vi "NewCombined.vi"() -> ()   [LabVIEW 2020]
uses:
  Stage/New/StageOptions.ctl
  Stage/New/SettingCtrlOptions.ctl
  Stage/New/PosCtrlOptions.ctl
  Stage/libximc.lvlib
  <instrlib>/_niInstr/Basic Elements/v1/FPGA/niInstr Basic Elements v1 FPGA.lvlib
  Digi/Digitizer_StatesMain.ctl
  Digi/SubVIs/DigiFPGARef.ctl
  <vilib>/rvi/interface/nirviMethod/nirviMethod.xnode
  <vilib>/FPGAPlugInAG/Dynamic/niLvFpga_Reset_Dynamic.vi
  <vilib>/rvi/interface/nirviReadWriteControl/nirviReadWriteControl.xnode
  NiFpgaLv.dll
  <vilib>/Utility/error.llb/Error Cluster From Error Code.vi
  <vilib>/rvi/interface/Simulation/niFpgaSimulationCallBeginRW.vi
  <vilib>/rvi/errors/niLvFpgaAdjustHostInterfaceError.vi
  <vilib>/rvi/interface/nirviCloseFPGA/nirviCloseFPGA.xnode
  <vilib>/FPGAPlugInAG/Dynamic/niLvFpga_Close_Dynamic.vi
  Gen/Generator_States.ctl
  ScanStates_main.ctl
  <vilib>/UPVI/lvhdf5/file.llb/LVH5F Operation.ctl
  <vilib>/UPVI/lvhdf5/dataset.llb/LVH5D Operation.ctl
  <vilib>/UPVI/lvhdf5/library.llb/HDF5 Ref.ctl
  <vilib>/Utility/miscctls.llb/LVRectTypeDef.ctl
  <vilib>/UPVI/lvhdf5/identifier.llb/Not an HDF5 Refnum Constant.vi
  <vilib>/UPVI/lvhdf5/dataset.llb/Simple H5Dwrite (Variant).vi
  <vilib>/UPVI/lvhdf5/dataset.llb/OpenCreateReplace Dataset by Element Type.vi
  <vilib>/UPVI/lvhdf5/dataspace.llb/H5Sselect_hyperslab.vi
  <vilib>/UPVI/lvhdf5/dataset.llb/H5Dwrite (Variant).vi
  <vilib>/UPVI/lvhdf5/dataset.llb/H5Dget_space.vi
  <vilib>/UPVI/lvhdf5/attribute.llb/private/LVH5AwriteWDTAttrs.vi
  <vilib>/UPVI/lvhdf5/dataspace.llb/H5Sclose.vi
  <vilib>/UPVI/lvhdf5/group.llb/H5G_obj_t.ctl
  <vilib>/UPVI/lvhdf5/utility.llb/Select HDF5 Dialog.vi
  <vilib>/UPVI/lvhdf5/dataset.llb/Simple H5Dwrite.xnode
  <vilib>/UPVI/lvhdf5/dataset.llb/Append Element(s) to Dataset (Variant).vi
  <vilib>/UPVI/lvhdf5/dataset.llb/Append Element(s) to Dataset.xnode
  <instrlib>/_niInstr/Basic Elements/v1/FPGA/Private/Count Up U32.vi
  <vilib>/UPVI/lvhdf5/utility.llb/Select HDF5 Dialog (File and Object).vi
  <vilib>/UPVI/lvhdf5/utility.llb/Select HDF5 Dialog (Object Only).vi
  FileStore/H5_WriteAttr.vi
  Digi/Controls/FPGA VI Reference.ctl
  <vilib>/userdefined/High Color/nirio_resource_hc.ctl
panel:
  out "Gen State":T1
  in  "Send vi Trig":bool
  in  "Generator Resource":refnum<k15>
  in  "Use Default Wave Settings":bool caption="Checkbox"
  in  "Stop Generator \nApplication":bool
  out "Gain":dbl
  out "Offset Factor":dbl
  out "Amplitudes":dbl[](array[numeric]) format="%.2f"
  out "Sampling Frequency (Hz)":u64
  out "Waves per Pixel":u32
  in  "Ext/nViTrig":bool=TRUE
  out "Gen Actual Sample Rate":dbl format="%#_6p"
  in  "Start Gen":bool
  in  "stop Gen":bool
  out "Generator On":bool
  out "Input Waveform":dbl[](graph)
  out "Intensity Graph":dbl[][](graph)
  in  "File Directory":path
  in  "Filename":string
  in  "Start Scan":bool
  in  "TrigIn_Sim":bool caption="Pause"
  in  "Delay(us)":sgl min=0 step=0.1 format="%#_4g"
  in  "Record Size":u16=1024
  in  "Time Division":u8(slide)=1 max=2 step=1 scale=0.0..2.0
  in  "Amplitude \nAveraging":u16(slide)=1 caption="Amplitude Averaging" scale=0.0..8.0 scale format="%#.2g"
  out "Configured?":bool
  out "TIS Configured?":bool
  in  "Start Digi":bool
  out "Digitizer On":bool
  in  "FineDelay  Control":dbl(slide)=1.0 scale=-2.0..2.0
  in  "Amplitude Range":cluster{"Slider 1":dbl, "Slider 1":dbl}(slide)={"Slider 1"=1.0, "Slider 1"=1.6299559471365639} scale=-2.5..2.5
  in  "Range":dbl=2.0
  out "Waveform LIVE":cluster{"Start Time":dbl, dbl, ext[]}(graph)
  out "Trigger Count":u32
  in  "reset":bool
  out "count out":u32
  out "Trig In":u32
  in  "Trigger Type":enum8{"Software", "Data Edge"}(ring)
  out "AvgCount_powerOf2":u16(knob) caption="Amplitude Avg" max=8 step=1 scale=0.0..8.0
  out "WaveSampleCount":i16=1024
  in  "Trigger Level (V)":dbl
  out "Read Size (Host)":u16
  out "TimeDivFactor":i16
  out "FPGA VI Reference Out":T2
  out "range (Vpp)":dbl=1.3
  out "Digi State":T3
  in  "Machine Mode":T4(ring)=enum."Normal"
  in  "nGenTrig/vi":bool=TRUE caption="Trigger Mode"
  in  "Digi RIO Resource":T5="PXI1Slot2"
  in  "Stop Digi App":bool caption="Stop Digi \nApplication"
  out "Moving?":bool
  out "Stage Position":cluster{sgl[], sgl[]}(graph) caption="XY Graph - Dark"
  in  "X Position Abs":dbl caption="X Position"
  in  "Y Position Abs":dbl caption="Y Position"
  out "Line Count":i32=6
  out "Pixel Count":i32=6
  in  "X Start":sgl
  in  "X End":sgl=10.0
  in  "Y Start":sgl
  in  "Y End":sgl=8.0
  in  "Y Step Size 2":sgl=0.5
  in  "X Step Size 2":sgl=0.5
  in  "Scan Mode":enum16{"Raster", "Serpentine"}(ring)
  out "X Step Size":sgl format="%#.2g"
  out "Y Step Size":sgl format="%#.2g"
  in  "Speed Control (mm/s)":sgl(slide)=1.0 min=0.1 scale=0.1..5.0
  in  "AbsMove":bool
  in  "Outline":bool
  in  "Start Stage":bool
  in  "Stop Motion":bool
  in  "Zero":bool
  in  "Right":bool
  in  "Left":bool
  in  "Move to Start":bool
  in  "Down":bool
  in  "Up":bool
  out "X Position":dbl format="%#.3g"
  out "Y Position":dbl format="%#.3g"
  in  "Move Step":dbl=1.0
  in  "Stop Stage":bool
  out "Controller Open?":bool
  in  "Next Coordinate Index":i32
  out "Coordinate Array":sgl[][](array[numeric])
  out "Step Sizes":sgl[](array[numeric])
  out "Peripheral Coordis":sgl[][](array[numeric])=[[0.0, 0.0], [1.8, 0.0], [3.6, 0.0], [5.3999996, 0.0], [7.2, 0.0], [9.0, 0.0], [9.0, 2.0], [7.2, 2.0], [5.3999996, 2.0], [3.6, 2.0], [1.8, 2.0], [0.0, 2.0], [0.0, 4.0], [1.8, 4.0], [3.6, 4.0], [5.3999996, 4.0], [7.2, 4.0], [9.0, 4.0], [9.0, 6.0], [7.2, 6.0], [5.3999996, 6.0], [3.6, 6.0], [1.8, 6.0], [0.0, 6.0], [0.0, 8.0], [1.8, 8.0], [3.6, 8.0], [5.3999996, 8.0], [7.2, 8.0], [9.0, 8.0], [9.0, 10.0], [7.2, 10.0], [5.3999996, 10.0], [3.6, 10.0], [1.8, 10.0], [0.0, 10.0]]
  out "Serial nos":u32[](array[numeric])
  out "Calibration":cluster{dbl, "MicrostepMode":u32}[](array[cluster])
  out "IDs":i32[](array[numeric])
  out "Move Step halved":dbl=1.0
  out "X Max Stage":dbl=220.0 format="%#_13g"
  out "Y Maximum":dbl
  in  "Correction Table Path (Hidden)":path
  in  "EdgePt/nPixelMap":bool=TRUE
  out "Stage Status":T6
  in  "Close Stage":bool
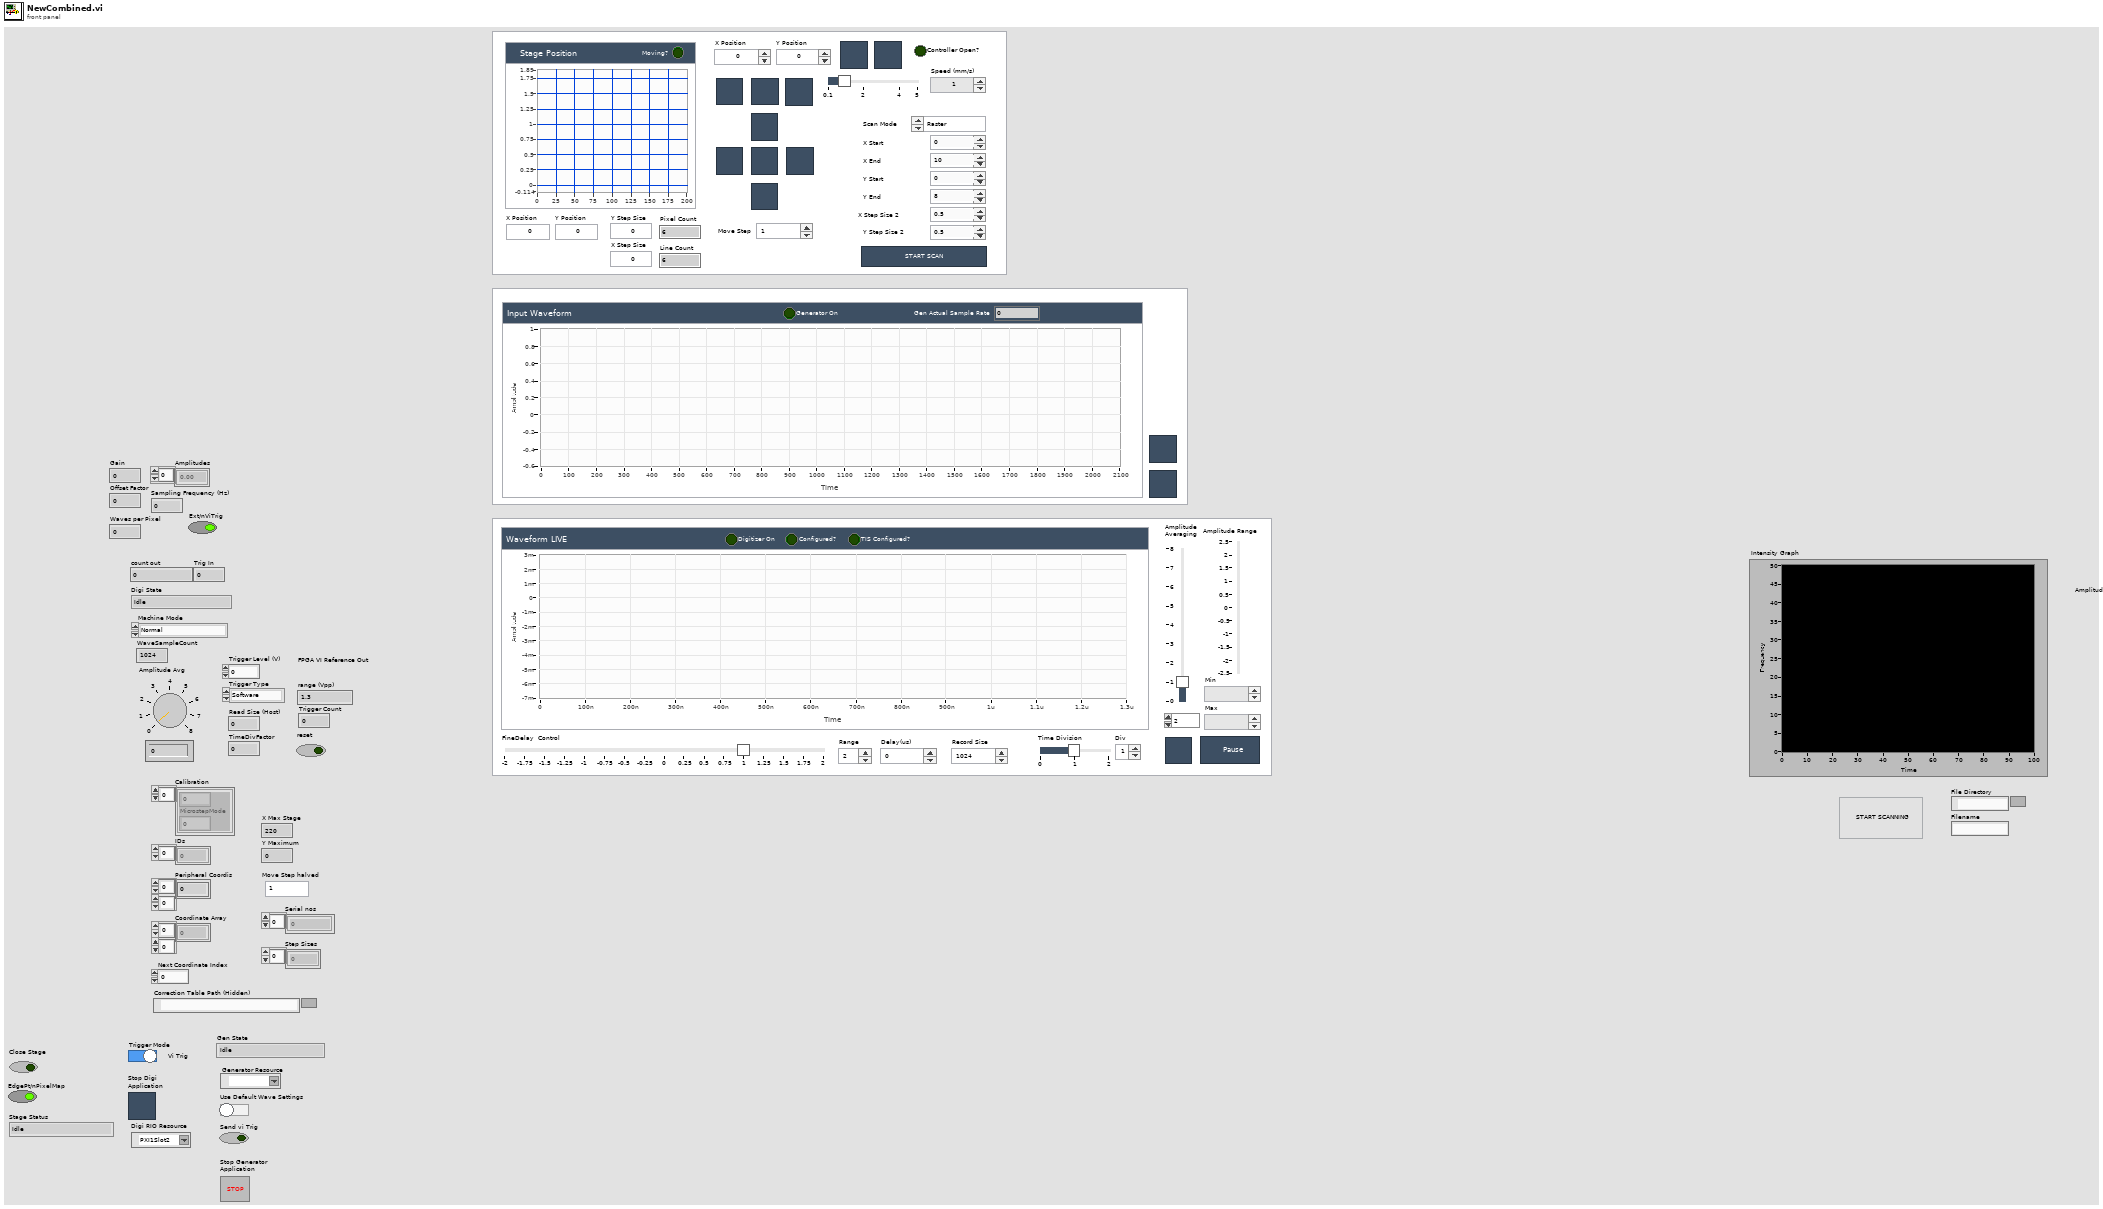
[diagram p1: front panel]
types:
  T1 = typedef "Generator_States.ctl" = enum16{"Idle", "GenerateWaveArray", "InitGen", "SendVITrig", "CloseGen", "CloseApp"}
  T2 = typedef "DigiFPGARef.ctl" = refnum<k20>
  T3 = typedef "Digitizer_StatesMain.ctl" = enum16{"Idle", "Init", "SetParam", "VITrig", "Read", "CloseDigi", "CloseApp"}
  T4 = enum16{"Scanning Mode", "Perimeter Mode", "Normal"}
  T5 = typedef "nirio_resource_hc.ctl" = tag
  T6 = typedef "StageOptions.ctl" = enum16{"Idle", "Init", "Set Speed", "GenerateMotionPoints", "Scan_Start", "Scan_MoveNext", "Scan_SyncSet", "Scan_Get Pos", "Scan_Complete", "Cmd_MoveAbs", "Cmd_CloseControllers", "Cmd_MoveUp", "Cmd_MoveDown", "Cmd_MoveLeft", "Cmd_MoveRight", "Cmd_MoveStart", "Cmd_MoveZero", "Cmd_GetPos", "Cmd_Stop", "Sync_On", "Sync_Off", "Stop Motion", "CloseApplication"}
  T7 = typedef "ScanStates_main.ctl" = enum16{"Idle", "Init", "Get Data", "Store Data", "Close Files"}
  T8 = typedef "SettingCtrlOptions.ctl" = enum16{"Set X", "Set Y", "Set X and Y", "Get Settings", "None"}
  T9 = typedef "PosCtrlOptions.ctl" = enum16{"Move X", "Move Y", "Both X and Y", "Read Pos", "None"}
  T10 = typedef "FPGA VI Reference.ctl" = refnum<k20>
  T11 = typedef "LVH5D Operation.ctl" = enum16{"open", "replace", "create", "open or create", "create or replace", "create or replace with confirmation"}
  T12 = typedef "LVH5F Operation.ctl" = enum16{"open", "open or create", "create or replace", "create or replace (with confirmation)", "create", "open (read only)"}
  T13 = typedef "LVRectTypeDef.ctl" = cluster{"Left":i16, "Top":i16, "Right":i16, "Bottom":i16}
  T14 = cluster{"Behavior":enum32{"Invalid", "Default", "Floating", "Floating/Auto-Hide", "Modal"}, "Position":T13, "Center":bool, "Title":string}
  T15 = typedef "H5G_obj_t.ctl" = i32
  T16 = cluster{"Object Types (any)":T15[], "Object Pattern":string}
  T17 = typedef "HDF5 Ref.ctl" = refnum<k1>
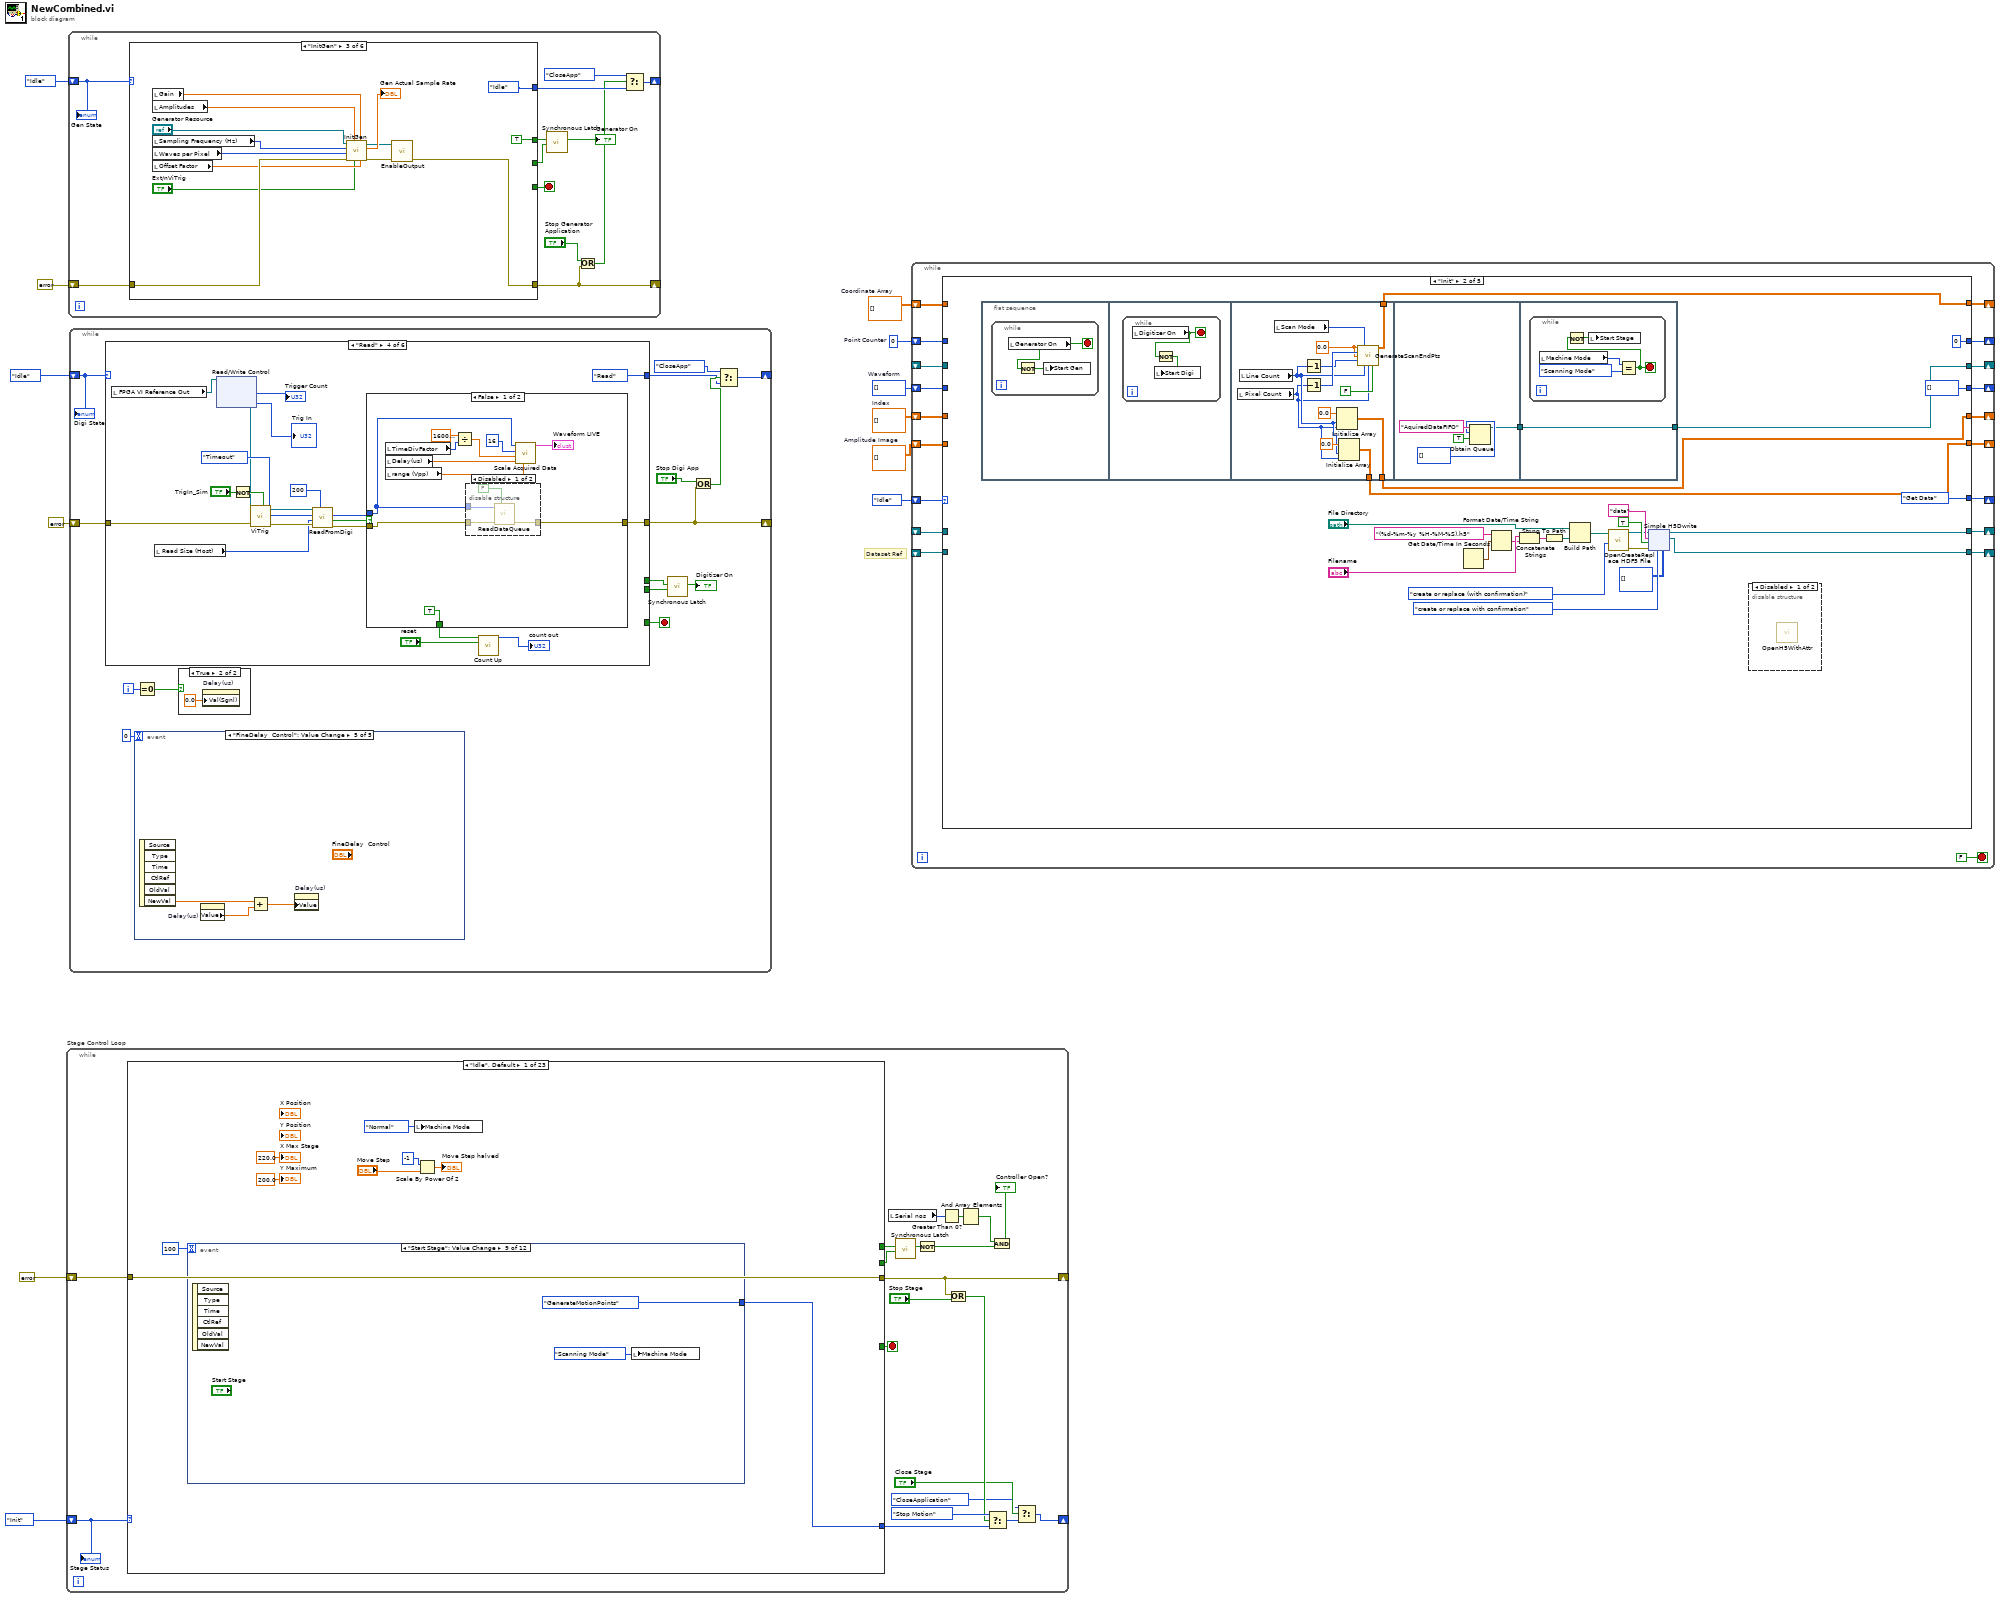
[diagram p0: block diagram]
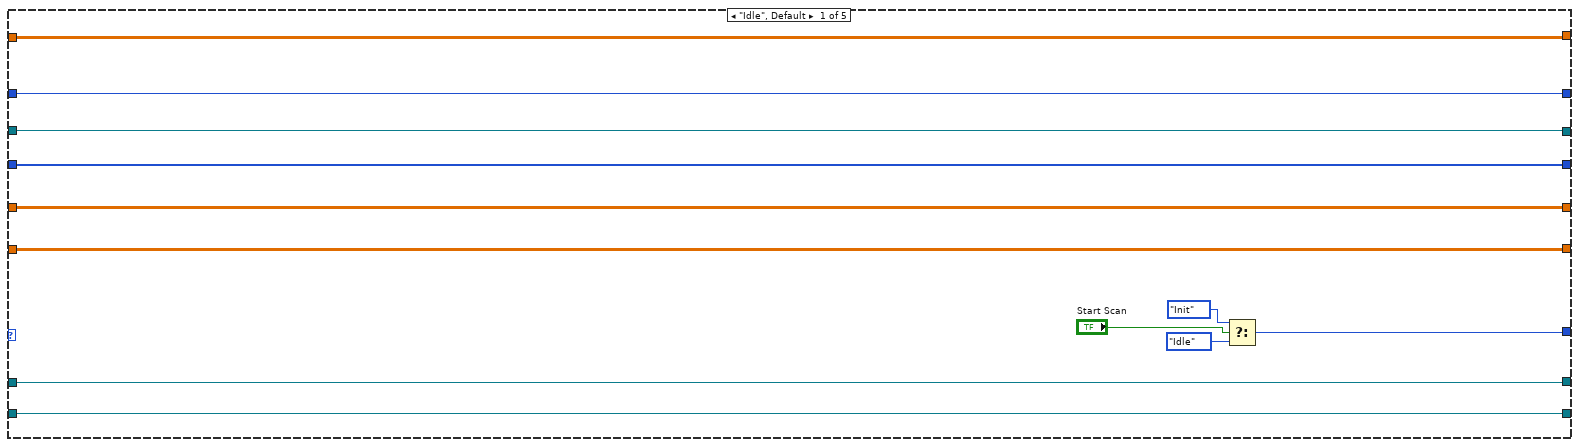
[diagram p2: hidden frame]
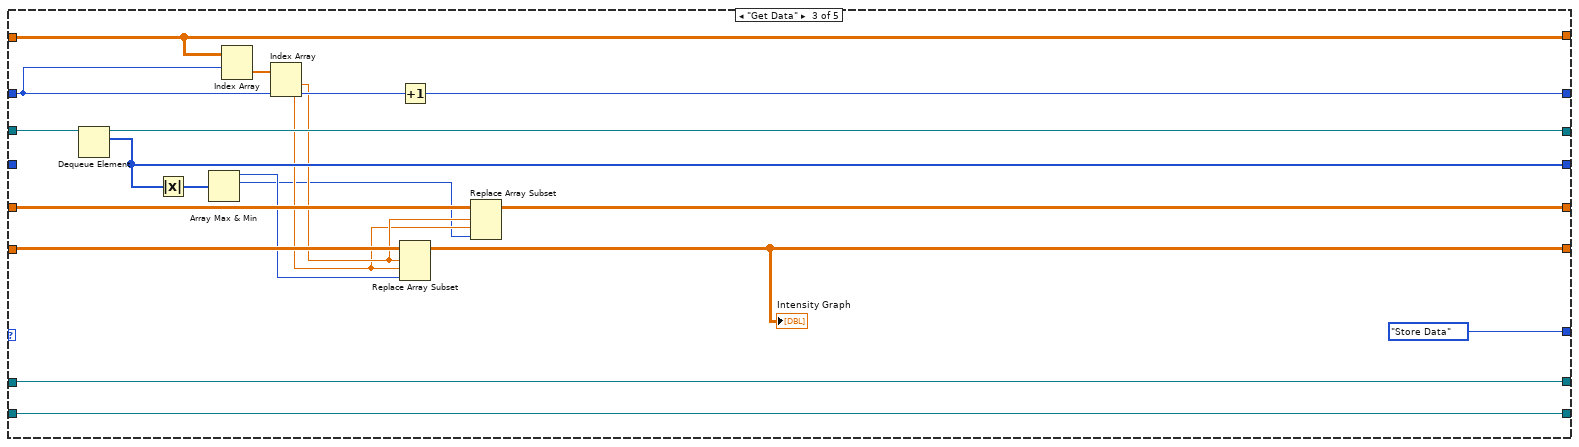
[diagram p4: hidden frame]
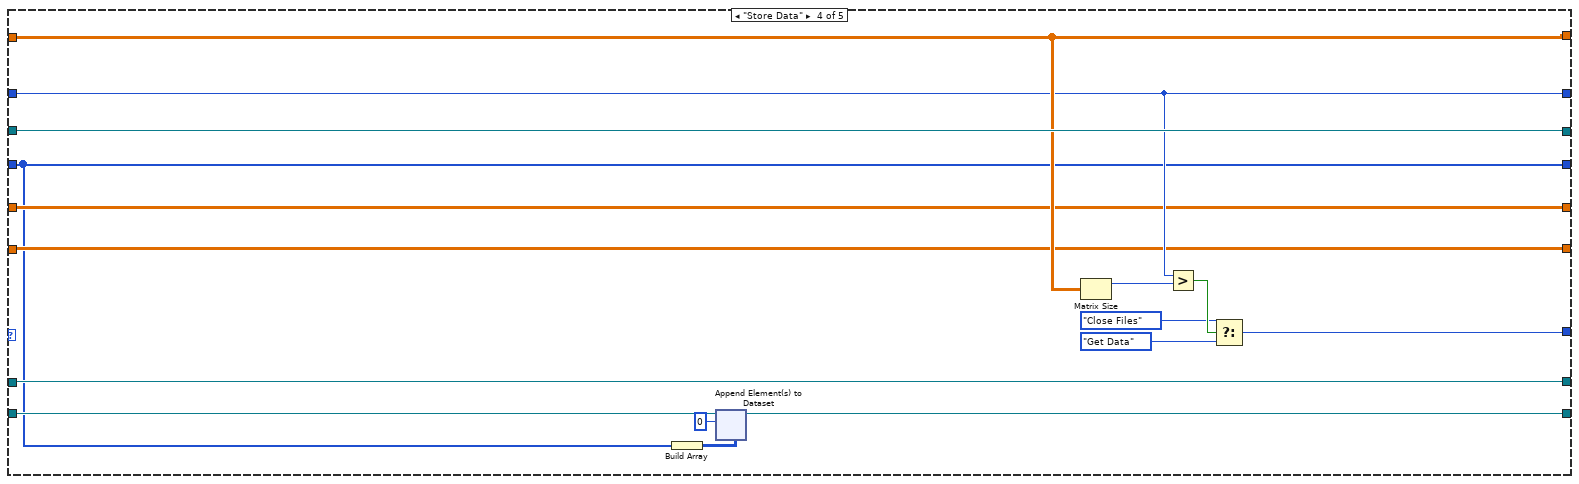
[diagram p5: hidden frame]
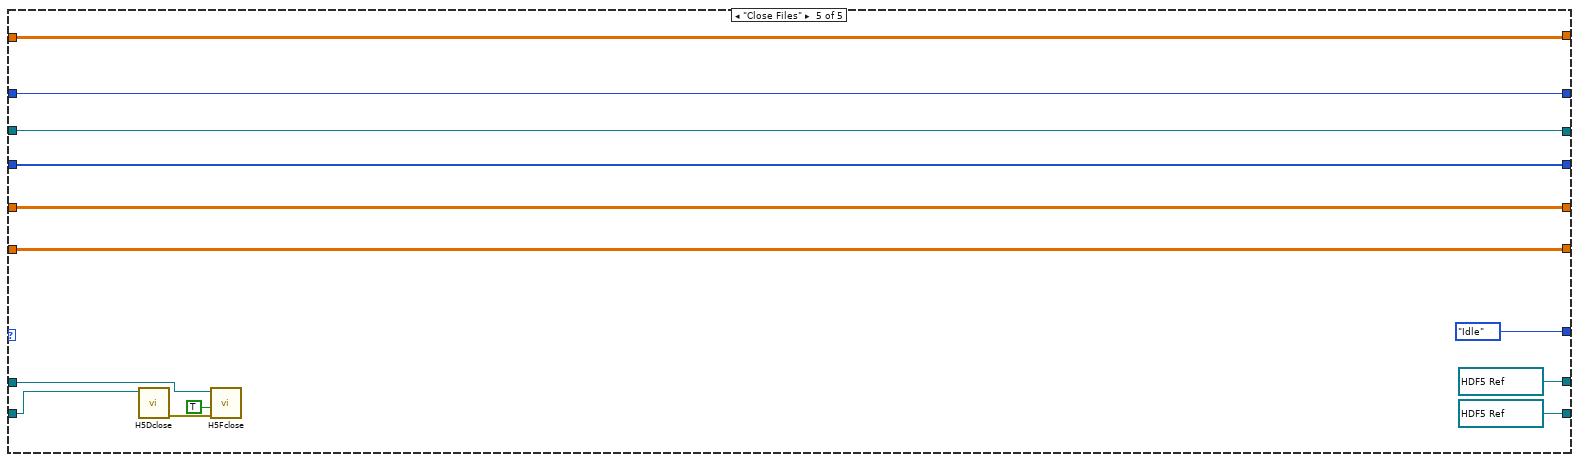
[diagram p6: hidden frame]
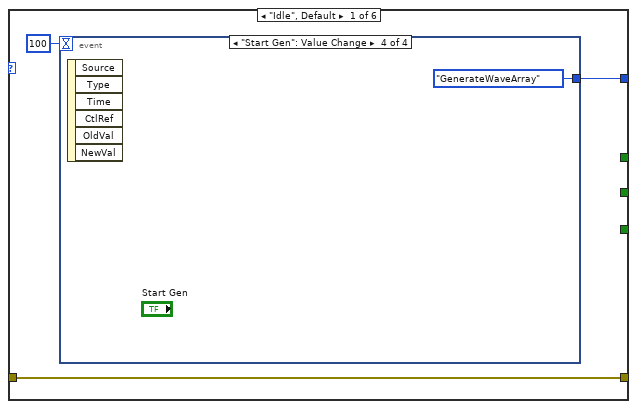
[diagram p7: hidden frame]
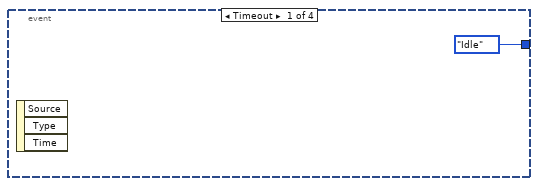
[diagram p8: hidden frame]
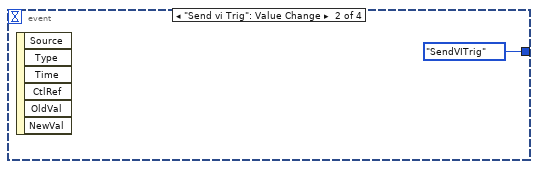
[diagram p9: hidden frame]
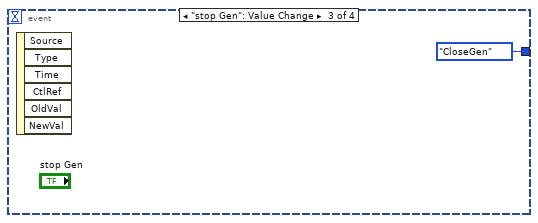
[diagram p10: hidden frame]
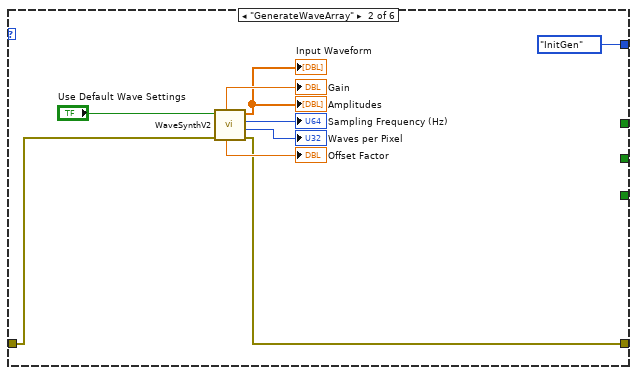
[diagram p11: hidden frame]
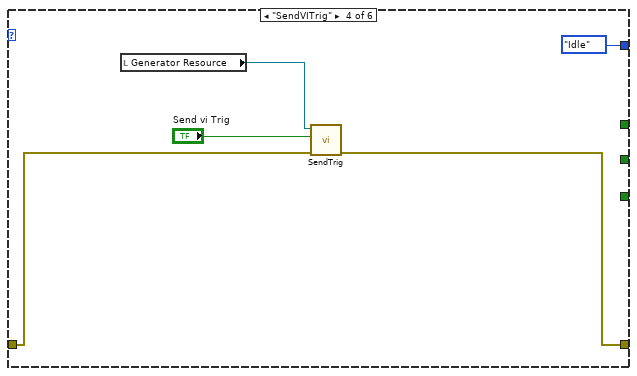
[diagram p12: hidden frame]
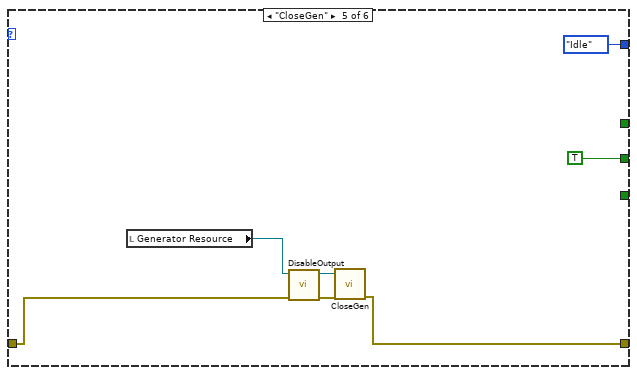
[diagram p13: hidden frame]
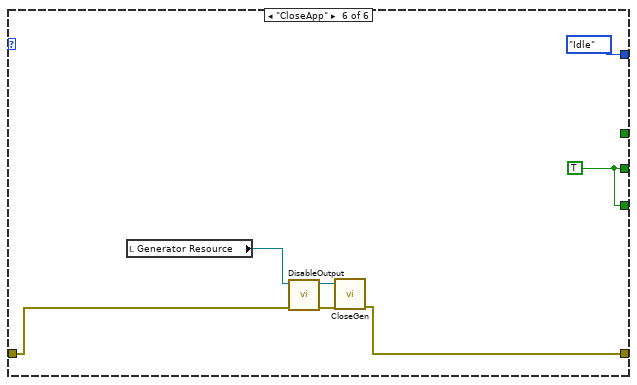
[diagram p14: hidden frame]
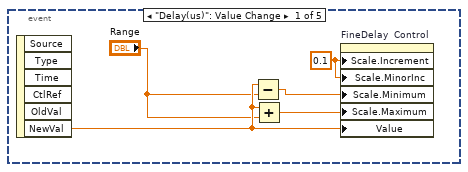
[diagram p15: hidden frame]
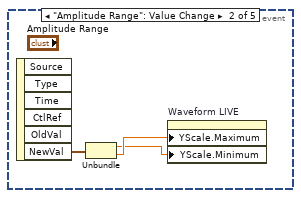
[diagram p16: hidden frame]
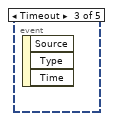
[diagram p17: hidden frame]
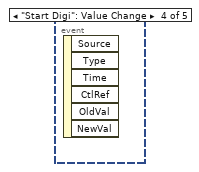
[diagram p18: hidden frame]
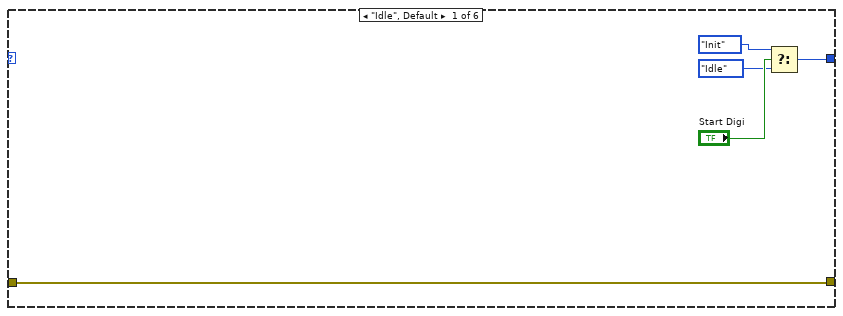
[diagram p20: hidden frame]
diagram:
  w6 = dbl[][] []  # Index
  w5 = dbl[][] []  # Amplitude Image
  w4 = i16[] []  # Waveform
  w3 = sgl[][] []  # Coordinate Array
  w2 = u64 0  # Point Counter
  # "Dataset Ref"
  n1 = while "Stage Control Loop" {
    shift-right: [w21] -> _
    shift-left: StageOptions."Init" -> [w32]
    shift-right: [w29] -> _
    shift-left: errorcluster {"status"=FALSE, "code"=0, "source"=""} ("error out") -> [w30]
    stop <- w22 stop-if-true
    n2 = case shown="\"Idle\", Default" w32 {
      tunnel: [w41 w82 w105 w134 w148 w180 w194 w207 w248 w257 w266 w273 w284 w294 w304 w313 w321 w336 w342 w353 w362 w369 w379] -> w29
      tunnel: w30 -> [w41 w89 w106 w133 w154 w181 w195 w208 w249 w258 w267 w272 w285 w295 w305 w314 w322 w337 w341 w354 w363 w368 w378]
      tunnel: [w40 StageOptions."Set Speed" StageOptions."Idle" w114 StageOptions."Scan_Get Pos" w169 StageOptions."Scan_MoveNext" w204 StageOptions."Idle" StageOptions."Idle" StageOptions."Idle" StageOptions."Idle" StageOptions."Idle" StageOptions."Idle" StageOptions."Idle" StageOptions."Idle" StageOptions."Idle" StageOptions."Idle" StageOptions."Idle" StageOptions."Idle" StageOptions."Idle" StageOptions."Idle" StageOptions."Idle"] -> w27
      tunnel: [_ _ _ _ _ _ _ _ _ _ _ _ _ _ _ _ _ _ _ _ _ w365 w374] -> w25
      tunnel: [_ w83 _ _ _ _ _ _ _ _ _ _ _ _ _ _ _ _ _ _ _ _ _] -> w23
      tunnel: [_ _ _ _ _ _ _ _ _ _ _ _ _ _ _ _ _ _ _ _ _ _ w374] -> w22
      frame "Idle", Default {
        n3 = event shown="[8] \"Start Stage\": Value Change" {
          selector: _ -> [_ _ _ _ _ _ _ _ _ _ _ _]
          dyn-events: _ -> [_ _ _ _ _ _ _ _ _ _ _ _]
          timeout: 100 -> [_ _ _ _ _ _ _ _ _ _ _ _]
          tunnel: [w42 StageOptions."Cmd_MoveUp" StageOptions."Cmd_MoveDown" StageOptions."Cmd_MoveStart" StageOptions."Cmd_MoveLeft" StageOptions."Cmd_MoveRight" StageOptions."Cmd_MoveZero" StageOptions."Cmd_Stop" StageOptions."GenerateMotionPoints" StageOptions."Set Speed" w77 StageOptions."Cmd_MoveAbs"] -> w40
          event Timeout {
            n4 = event-data() -> ()  [unwired: 1 in, 3 out]
            n5 = local read "Controller Open?"() -> (w43:bool)
            n6 = case shown="True" w43 {
              tunnel: [StageOptions."Init" StageOptions."Cmd_GetPos"] -> w42
              frame False {
              }
              frame True {
              }
            }
          }
          event "Up": Value Change {
            w48 = 0.0 ("X Scale.Range:Minimum")
            n7 = event-data() -> ()  [unwired: 1 in, 6 out]
            n8 = local read "X Max Stage"() -> (w47:dbl)
            n9 = local read "Y Maximum"() -> (w46:dbl)
            n10 = Build Array(w48, w47) -> (w50:dbl[])
            n11 = Build Array(w48, w46) -> (w49:dbl[])
            n12 = property on="Stage Position" class="XYGraph (strict)"("XScale.Maximum"=w47, "XScale.Minimum"=w48, "YScale.Maximum"=w46, "YScale.Minimum"=w48, "XScale.MarkerVals[]"=w50, "YScale.MarkerVals[]"=w49) -> ()  [unwired: 2 in, 2 out]
          }
          event "Down": Value Change {
            w54 = 0.0 ("X Scale.Range:Minimum")
            n13 = event-data() -> ()  [unwired: 1 in, 6 out]
            n14 = local read "X Max Stage"() -> (w53:dbl)
            n15 = local read "Y Maximum"() -> (w52:dbl)
            n16 = Build Array(w54, w53) -> (w56:dbl[])
            n17 = Build Array(w54, w52) -> (w55:dbl[])
            n18 = property on="Stage Position" class="XYGraph (strict)"("XScale.Maximum"=w53, "XScale.Minimum"=w54, "YScale.Maximum"=w52, "YScale.Minimum"=w54, "XScale.MarkerVals[]"=w56, "YScale.MarkerVals[]"=w55) -> ()  [unwired: 2 in, 2 out]
          }
          event "Move to Start": Value Change {
            n19 = event-data() -> ()  [unwired: 1 in, 6 out]
          }
          event "Left": Value Change {
            w61 = 0.0 ("X Scale.Range:Minimum")
            n20 = event-data() -> ()  [unwired: 1 in, 6 out]
            n21 = local read "X Max Stage"() -> (w60:dbl)
            n22 = local read "Y Maximum"() -> (w59:dbl)
            n23 = Build Array(w61, w60) -> (w63:dbl[])
            n24 = Build Array(w61, w59) -> (w62:dbl[])
            n25 = property on="Stage Position" class="XYGraph (strict)"("XScale.Maximum"=w60, "XScale.Minimum"=w61, "YScale.Maximum"=w59, "YScale.Minimum"=w61, "XScale.MarkerVals[]"=w63, "YScale.MarkerVals[]"=w62) -> ()  [unwired: 2 in, 2 out]
          }
          event "Right": Value Change {
            w65 = 0.0 ("X Scale.Range:Minimum")
            n26 = event-data() -> ()  [unwired: 1 in, 6 out]
            n27 = local read "X Max Stage"() -> (w67:dbl)
            n28 = local read "Y Maximum"() -> (w66:dbl)
            n29 = Build Array(w65, w67) -> (w69:dbl[])
            n30 = Build Array(w65, w66) -> (w68:dbl[])
            n31 = property on="Stage Position" class="XYGraph (strict)"("XScale.Maximum"=w67, "XScale.Minimum"=w65, "YScale.Maximum"=w66, "YScale.Minimum"=w65, "XScale.MarkerVals[]"=w69, "YScale.MarkerVals[]"=w68) -> ()  [unwired: 2 in, 2 out]
          }
          event "Zero": Value Change {
            n32 = event-data() -> ()  [unwired: 1 in, 6 out]
          }
          event "Stop Motion": Value Change {
            n33 = event-data() -> ()  [unwired: 1 in, 6 out]
          }
          event "Start Stage": Value Change {
            n34 = event-data() -> ()  [unwired: 1 in, 6 out]
            n35 = local write "Machine Mode"(T4."Scanning Mode" ("Machine Mode")) -> ()
          }
          event "Speed Control (mm/s)": Value Change {
            n36 = event-data() -> ()  [unwired: 1 in, 6 out]
          }
          event "Outline": Value Change {
            n37 = event-data() -> ()  [unwired: 1 in, 6 out]
            n38 = case shown="False" "Outline" {
              tunnel: [StageOptions."Idle" StageOptions."GenerateMotionPoints"] -> w77
              frame False {
              }
              frame True {
                n39 = local write "Machine Mode"(T4."Perimeter Mode" ("Machine Mode")) -> ()
              }
            }
          }
          event "AbsMove": Value Change {
            n40 = event-data() -> ()  [unwired: 1 in, 6 out]
          }
        }
        n41 = local write "Machine Mode"(T4."Normal" ("Machine Mode")) -> ()
        n42 = Scale By Power Of 2(n=i16 -1, x="Move Step") -> (x*2^n=→"Move Step halved":dbl)
        "X Max Stage" <- 220.0 ("X Max Stage")
        "Y Maximum" <- 200.0 ("Y Maximum")
      }
      frame "Init" {
        w90 = 100  # numSteps = 1mm
        w91 = TRUE  # Correction File Path Option
        n43 = case shown="False" w91 {
          tunnel: ["Correction Table Path (Hidden)" w97] -> w92
          frame False {
          }
          frame True {
            w98 = path "Corr_table_8MT173-25.tbl"  # File Name
            n44 = Current VI's Path() -> (path=w100:path)
            n45 = Build Path(base path=w100, name or relative path=path "") -> (appended path=w99:path)
            n46 = Build Path(base path=w99, name or relative path=w98) -> (appended path=w97:path)
          }
        }
        n47 = call "Find Controllers.vi"("error in (no error)"=w89) -> ("error out"=w94:errorcluster, "Names"=w95:string[])  [unwired: 8 in, 1 out]
        n48 = call "OpenDevices.vi"("error In"=w94, "Names"=w95) -> ("error out"=w93:errorcluster, "Serial nos"=→"Serial nos":u32[], "IDs"=w87:i32[])  [unwired: 6 in]
        "IDs" <- w87
        n49 = call "CalibrateStage.vi"("error in (no error)"=w93, "numSteps = 1mm"=w90, "Correction Table Path"=w92, "IDs"=w87) -> ("error out"=w82:errorcluster, "Calibration"=→"Calibration":cluster{dbl, "MicrostepMode":u32}[])  [unwired: 2 in, 4 out]
        n50 = Unbundle By Name(w82) -> ("status"=w84:bool)
        n51 = Not(x=w84) -> (.not. x?=w83:bool)
      }
      frame "Set Speed" {
        n52 = local read "IDs"() -> (w104:i32[])
        n53 = local read "Calibration"() -> (w103:cluster{dbl, "MicrostepMode":u32}[])
        n54 = call "SetMoveSettings.vi"("Mode"=SettingCtrlOptions."Set X and Y", "error in (no error)"=w106, "Calibration"=w103, "Speed"="Speed Control (mm/s)", "IDs"=w104) -> ("error out"=w105:errorcluster)  [unwired: 4 in, 2 out]
      }
      frame "GenerateMotionPoints" {
        n55 = local read "Calibration"() -> (w120:cluster{dbl, "MicrostepMode":u32}[])
        n56 = Subtract(x="X End", y="X Start") -> (x-y=w130:sgl)
        n57 = Increment(x=w130) -> (x+1=w129:sgl)
        n58 = Divide(x=w129, y="X Step Size 2") -> (x/y=w127:sgl)
        n59 = To Long Integer(number=w127) -> (32bit integer=w126:i32)
        "Pixel Count" <- w126
        n60 = Subtract(x="Y End", y="Y Start") -> (x-y=w124:sgl)
        n61 = Increment(x=w124) -> (x+1=w125:sgl)
        n62 = Divide(x=w125, y="Y Step Size 2") -> (x/y=w122:sgl)
        n63 = To Long Integer(number=w122) -> (32bit integer=w121:i32)
        "Line Count" <- w121
        n64 = call "GenerateScanEndPts.vi"("X Start"="X Start", "Mode"="Scan Mode", "Calibration In"=w120, "X End"="X End", "Y Start"="Y Start", "Y End"="Y End", "error in"=w133, "Line Count"=w121, "Pixel Count"=w126, "EdgePt/nPixelMap"="EdgePt/nPixelMap") -> ("Coordinate Array"=→"Coordinate Array":sgl[][], "Step Sizes"=w111:sgl[], "error out"=w134:errorcluster)  [unwired: 1 in, 2 out]
        "Step Sizes" <- w111
        n65 = call "PeripheralCoordinates.vi"("Y End"="Y End", "Y Start"="Y Start", "X End"="X End", "X Start"="X Start") -> ("Coordinate Array"=→"Peripheral Coordis":sgl[][])  [unwired: 7 in]
        n66 = Index Array(array=w111) -> (element #1=→"X Step Size":sgl, element #2=→"Y Step Size":sgl)  [unwired: 2 in]
        n67 = case shown="\"Perimeter Mode\"" "Machine Mode" {
          tunnel: [StageOptions."Scan_Start" StageOptions."Scan_Start" StageOptions."Idle"] -> w114
          frame "Scanning Mode" {
          }
          frame "Perimeter Mode" {
          }
          frame "Normal", Default {
          }
        }
      }
      frame "Scan_Start" {
        w151 = 0.0 ("element")
        w160 = 1.0  # Offset
        # "Draw Markers To Indicate the Scan Area"
        n68 = property on="X End" class="DigNum (strict)"() -> ("Value"=w159:sgl)  [unwired: 2 in, 2 out]
        n69 = property on="X Start" class="DigNum (strict)"() -> ("Value"=w158:sgl)  [unwired: 2 in, 2 out]
        n70 = property on="Y End" class="DigNum (strict)"() -> ("Value"=w155:sgl)  [unwired: 2 in, 2 out]
        n71 = property on="Y Start" class="DigNum (strict)"() -> ("Value"=w157:sgl)  [unwired: 2 in, 2 out]
        n72 = Add(x=w160, y=w159) -> (x+y=w162:dbl)
        n73 = Subtract(x=w158, y=w160) -> (x-y=w163:dbl)
        n74 = Add(x=w155, y=w160) -> (x+y=w161:dbl)
        n75 = Subtract(x=w157, y=w160) -> (x-y=w156:dbl)
        n76 = Build Array(w158, w159) -> (w165:sgl[])
        n77 = Build Array(w157, w155) -> (w164:sgl[])
        n78 = property on="Stage Position" class="XYGraph (strict)"(error in=w154, "XScale.Maximum"=w162, "XScale.Minimum"=w163, "YScale.Maximum"=w161, "YScale.Minimum"=w156, "XScale.MarkerVals[]"=w165, "YScale.MarkerVals[]"=w164) -> (error out=w140:errorcluster)  [unwired: 1 in, 1 out]
        n79 = local read "EdgePt/nPixelMap"() -> (w144:bool)
        n80 = local read "IDs"() -> (w147:i32[])
        n81 = local read "Step Sizes"() -> (w145:sgl[])
        n82 = local read "Calibration"() -> (w146:cluster{dbl, "MicrostepMode":u32}[])
        n83 = call "SetSyncSettings.vi"("Periodic/nPointScan"=w144, "X SyncOut Enabled"=FALSE, "Y SyncOut Enabled"=FALSE, "error in (no error)"=w140, "Calibration"=w146, "Step Sizes(mm)"=w145, "IDs"=w147) -> ("error out"=w141:errorcluster)  [unwired: 3 in, 1 out]
        n84 = local write "Next Coordinate Index"(0 ("Next Coordinate Index")) -> ()
        n85 = local read "IDs"() -> (w149:i32[])
        n86 = local read "Calibration"() -> (w150:cluster{dbl, "MicrostepMode":u32}[])
        n87 = Build Array(w151, w151) -> (w152:dbl[])
        n88 = call "PositionControlRelative.vi"("Mode"=PosCtrlOptions."Both X and Y", "error in (no error)"=w141, "Calibration"=w150, "Move to"=w152, "IDs"=w149) -> ("error out"=w148:errorcluster)  [unwired: 4 in, 2 out]
      }
      frame "Scan_Get Pos" {
        n89 = local read "IDs"() -> (w178:i32[])
        n90 = local read "Calibration"() -> (w179:cluster{dbl, "MicrostepMode":u32}[])
        n91 = call "PositionControl.vi"("Mode"=PosCtrlOptions."Read Pos", "error in (no error)"=w181, "Calibration"=w179, "IDs"=w178) -> ("error out"=w180:errorcluster, "Moving?"=w168:bool, "Position"=w171:sgl[])  [unwired: 4 in, 1 out]
        n92 = local write "Moving?"(w168) -> ()
        n93 = Index Array(array=w171, index #1=0 ("index"), index #2=1 ("index")) -> (element #1=w175:sgl, element #2=w174:sgl)
        n94 = local write "X Position"(w175) -> ()
        n95 = local write "Y Position"(w174) -> ()
        n96 = Build Array(w175) -> (w176:sgl[])
        n97 = Build Array(w174) -> (w177:sgl[])
        n98 = Bundle(w176, w177) -> (w170:cluster{sgl[], sgl[]})  [unwired: 1 in]
        n99 = local write "Stage Position"(w170) -> ()
        n100 = Select(t=StageOptions."Scan_Get Pos", s=w168, f=StageOptions."Scan_SyncSet") -> (s? t:f=w169:T6)
      }
      frame "Scan_SyncSet" {
        n101 = local read "EdgePt/nPixelMap"() -> (w184:bool)
        n102 = local read "IDs"() -> (w192:i32[])
        n103 = local read "Step Sizes"() -> (w190:sgl[])
        n104 = local read "Calibration"() -> (w191:cluster{dbl, "MicrostepMode":u32}[])
        n105 = Quotient & Remainder(x="Next Coordinate Index", y=2) -> (x-y*floor(x/y)=w187:i32)  [unwired: 1 out]
        n106 = Not Equal To 0?(x=w187) -> (x != 0?=w185:bool)
        n107 = Compound Arithmetic op=OR(invert w184, w185) -> (w186:bool)
        n108 = call "SetSyncSettings.vi"("Periodic/nPointScan"=w184, "X SyncOut Enabled"=w186, "Y SyncOut Enabled"=FALSE, "error in (no error)"=w195, "Calibration"=w191, "Step Sizes(mm)"=w190, "IDs"=w192) -> ("error out"=w194:errorcluster)  [unwired: 3 in, 1 out]
      }
      frame "Scan_MoveNext" {
        n109 = flat-sequence {
          tunnel: w208 -> [w211]
          tunnel: [w211] -> w199
          tunnel: [w210] -> w198
          tunnel: [w209] -> w196
          tunnel: [w219] -> w206
          tunnel: [w216] -> w205
          tunnel: [w215] -> w201
          tunnel: w199 -> [w220]
          tunnel: w198 -> [w215]
          tunnel: [w214] -> w197
          tunnel: w196 -> [w214]
          tunnel: [w230] -> w200
          tunnel: [w231] -> w207
          tunnel: w197 -> [w223]
          tunnel: w201 -> [w227]
          tunnel: w205 -> [w228]
          tunnel: w206 -> [w231]
          frame #0 {
            n110 = local read "Machine Mode"() -> (w209:T4)
            n111 = case shown="\"Perimeter Mode\"" w209 {
              tunnel: [w212 w213] -> w210
              frame "Scanning Mode", Default {
                n112 = local read "Coordinate Array"() -> (w212:sgl[][])
              }
              frame "Perimeter Mode" {
                n113 = local read "Peripheral Coordis"() -> (w213:sgl[][])
              }
            }
          }
          frame #1 {
            n114 = local read "IDs"() -> (w218:i32[])
            n115 = local read "Next Coordinate Index"() -> (w216:i32)
            n116 = local read "Calibration"() -> (w217:cluster{dbl, "MicrostepMode":u32}[])
            n117 = Index Array(array=w215, index (row)=w216) -> (element=w221:sgl[])  [unwired: 1 in]
            n118 = call "PositionControl.vi"("Mode"=PosCtrlOptions."Both X and Y", "error in (no error)"=w220, "Calibration"=w217, "Move to"=w221, "IDs"=w218) -> ("error out"=w219:errorcluster)  [unwired: 3 in, 3 out]
          }
          frame #2 {
            n119 = Matrix Size(0:w227) -> (1:w226:i32)  [unwired: 1 out]
            n120 = Increment(x=w228) -> (x+1=w224:i32)
            n121 = Greater?(x=w224, y=w226) -> (0:w225:bool)
            n122 = case shown="True" w225 {
              selector: w225 -> [w232 _]
              tunnel: w224 -> [w233 w236]
              tunnel: [w233 w235] -> w229
              tunnel: [w232 w234] -> w230
              tunnel: w223 -> [_ w237]
              frame False {
              }
              frame True {
                n123 = case shown="\"Scanning Mode\", Default" w237 {
                  tunnel: w236 -> [w239 _]
                  tunnel: [w239 0] -> w235
                  tunnel: [TRUE ("x > y?") w241] -> w234
                  frame "Scanning Mode", Default {
                  }
                  frame "Perimeter Mode" {
                    n124 = local read "Outline"() -> (w242:bool)
                    n125 = Not(x=w242) -> (.not. x?=w241:bool)
                  }
                }
              }
            }
            n126 = local write "Next Coordinate Index"(w229) -> ()
          }
        }
        n127 = Select(t=StageOptions."Scan_Complete", s=w200, f=StageOptions."Scan_Get Pos") -> (s? t:f=w204:T6)
      }
      frame "Scan_Complete" {
        w246 = 0.0 ("element")
        n128 = local read "IDs"() -> (w244:i32[])
        n129 = local read "Calibration"() -> (w245:cluster{dbl, "MicrostepMode":u32}[])
        n130 = Build Array(w246, w246) -> (w247:dbl[])
        n131 = call "PositionControl.vi"("Mode"=PosCtrlOptions."Both X and Y", "error in (no error)"=w249, "Calibration"=w245, "Move to"=w247, "IDs"=w244) -> ("error out"=w248:errorcluster)  [unwired: 3 in, 3 out]
      }
      frame "Cmd_MoveAbs" {
        n132 = local read "IDs"() -> (w256:i32[])
        n133 = local read "Calibration"() -> (w255:cluster{dbl, "MicrostepMode":u32}[])
        n134 = Build Array("X Position Abs", "Y Position Abs") -> (w254:dbl[])
        n135 = call "PositionControl.vi"("Mode"=PosCtrlOptions."Both X and Y", "error in (no error)"=w258, "Calibration"=w255, "Move to"=w254, "IDs"=w256) -> ("error out"=w257:errorcluster)  [unwired: 3 in, 3 out]
      }
      frame "Cmd_MoveStart" {
        n136 = local read "X Start"() -> (w261:sgl)
        n137 = local read "Y Start"() -> (w260:sgl)
        n138 = local read "IDs"() -> (w265:i32[])
        n139 = local read "Calibration"() -> (w264:cluster{dbl, "MicrostepMode":u32}[])
        n140 = Build Array(w261, w260) -> (w263:sgl[])
        n141 = call "PositionControl.vi"("Mode"=PosCtrlOptions."Both X and Y", "error in (no error)"=w267, "Calibration"=w264, "Move to"=w263, "IDs"=w265) -> ("error out"=w266:errorcluster)  [unwired: 3 in, 3 out]
      }
      frame "Cmd_CloseControllers" {
        n142 = local read "IDs"() -> (w270:i32[])
        n143 = for {
          shift-right: [w277] -> w274
          shift-left: w272 -> [w276]
          tunnel: w270 -> [w275] mode=indexing
          n144 = call "command stop.vi"("error in (no error)"=w276, "id"=w275) -> ("error out"=w277:errorcluster)  [unwired: 8 in, 1 out]
        }
        n145 = call "CloseDevices.vi"("error in (no error)"=w274, "Close"=TRUE, "Ids"=w270) -> ("error out"=w273:errorcluster)  [unwired: 8 in]
      }
      frame "Cmd_MoveUp" {
        n146 = local read "Move Step halved"() -> (w281:dbl)
        n147 = local read "IDs"() -> (w280:i32[])
        n148 = local read "Calibration"() -> (w279:cluster{dbl, "MicrostepMode":u32}[])
        n149 = Build Array(0.0 ("element"), w281) -> (w283:dbl[])
        n150 = call "PositionControlRelative.vi"("Mode"=PosCtrlOptions."Move Y", "error in (no error)"=w285, "Calibration"=w279, "Move to"=w283, "IDs"=w280) -> ("error out"=w284:errorcluster)  [unwired: 4 in, 2 out]
      }
      frame "Cmd_MoveDown" {
        n151 = local read "Move Step halved"() -> (w291:dbl)
        n152 = local read "IDs"() -> (w289:i32[])
        n153 = local read "Calibration"() -> (w288:cluster{dbl, "MicrostepMode":u32}[])
        n154 = Negate(x=w291) -> (-x=w290:dbl)
        n155 = Build Array(0.0 ("element"), w290) -> (w293:dbl[])
        n156 = call "PositionControlRelative.vi"("Mode"=PosCtrlOptions."Move Y", "error in (no error)"=w295, "Calibration"=w288, "Move to"=w293, "IDs"=w289) -> ("error out"=w294:errorcluster)  [unwired: 4 in, 2 out]
      }
      frame "Cmd_MoveLeft" {
        n157 = local read "Move Step halved"() -> (w302:dbl)
        n158 = local read "IDs"() -> (w298:i32[])
        n159 = local read "Calibration"() -> (w299:cluster{dbl, "MicrostepMode":u32}[])
        n160 = Negate(x=w302) -> (-x=w301:dbl)
        n161 = Build Array(w301, 0.0 ("element")) -> (w303:dbl[])
        n162 = call "PositionControlRelative.vi"("Mode"=PosCtrlOptions."Move X", "error in (no error)"=w305, "Calibration"=w299, "Move to"=w303, "IDs"=w298) -> ("error out"=w304:errorcluster)  [unwired: 4 in, 2 out]
      }
      frame "Cmd_MoveRight" {
        n163 = local read "Move Step halved"() -> (w311:dbl)
        n164 = local read "IDs"() -> (w309:i32[])
        n165 = local read "Calibration"() -> (w308:cluster{dbl, "MicrostepMode":u32}[])
        n166 = Build Array(w311, 0.0 ("element")) -> (w312:dbl[])
        n167 = call "PositionControlRelative.vi"("Mode"=PosCtrlOptions."Move X", "error in (no error)"=w314, "Calibration"=w308, "Move to"=w312, "IDs"=w309) -> ("error out"=w313:errorcluster)  [unwired: 4 in, 2 out]
      }
      frame "Cmd_MoveZero" {
        w319 = 0.0 ("element")
        n168 = local read "IDs"() -> (w317:i32[])
        n169 = local read "Calibration"() -> (w318:cluster{dbl, "MicrostepMode":u32}[])
        n170 = Build Array(w319, w319) -> (w320:dbl[])
        n171 = call "PositionControl.vi"("Mode"=PosCtrlOptions."Both X and Y", "error in (no error)"=w322, "Calibration"=w318, "Move to"=w320, "IDs"=w317) -> ("error out"=w321:errorcluster)  [unwired: 3 in, 3 out]
      }
      frame "Cmd_GetPos" {
        n172 = local read "IDs"() -> (w334:i32[])
        n173 = local read "Calibration"() -> (w335:cluster{dbl, "MicrostepMode":u32}[])
        n174 = call "PositionControl.vi"("Mode"=PosCtrlOptions."Read Pos", "error in (no error)"=w337, "Calibration"=w335, "IDs"=w334) -> ("error out"=w336:errorcluster, "Moving?"=→"Moving?":bool, "Position"=w326:sgl[])  [unwired: 4 in, 1 out]
        n175 = Index Array(array=w326, index #1=0 ("index"), index #2=1 ("index")) -> (element #1=w330:sgl, element #2=w329:sgl)
        n176 = local write "X Position"(w330) -> ()
        n177 = local write "Y Position"(w329) -> ()
        n178 = Build Array(w330) -> (w332:sgl[])
        n179 = Build Array(w329) -> (w333:sgl[])
        n180 = Bundle(w332, w333) -> (→"Stage Position":cluster{sgl[], sgl[]})  [unwired: 1 in]
      }
      frame "Cmd_Stop" {
        n181 = local read "IDs"() -> (w340:i32[])
        n182 = for {
          shift-right: [w345] -> w342
          shift-left: w341 -> [w344]
          tunnel: w340 -> [w343] mode=indexing
          n183 = call "command stop.vi"("error in (no error)"=w344, "id"=w343) -> ("error out"=w345:errorcluster)  [unwired: 8 in, 1 out]
        }
      }
      frame "Sync_On" {
        n184 = local read "EdgePt/nPixelMap"() -> (w348:bool)
        n185 = local read "IDs"() -> (w351:i32[])
        n186 = local read "Step Sizes"() -> (w349:sgl[])
        n187 = local read "Calibration"() -> (w350:cluster{dbl, "MicrostepMode":u32}[])
        n188 = call "SetSyncSettings.vi"("Periodic/nPointScan"=w348, "X SyncOut Enabled"=TRUE, "Y SyncOut Enabled"=FALSE, "error in (no error)"=w354, "Calibration"=w350, "Step Sizes(mm)"=w349, "IDs"=w351) -> ("error out"=w353:errorcluster)  [unwired: 3 in, 1 out]
      }
      frame "Sync_Off" {
        n189 = local read "EdgePt/nPixelMap"() -> (w357:bool)
        n190 = local read "IDs"() -> (w360:i32[])
        n191 = local read "Step Sizes"() -> (w358:sgl[])
        n192 = local read "Calibration"() -> (w359:cluster{dbl, "MicrostepMode":u32}[])
        n193 = call "SetSyncSettings.vi"("Periodic/nPointScan"=w357, "X SyncOut Enabled"=FALSE, "Y SyncOut Enabled"=FALSE, "error in (no error)"=w363, "Calibration"=w359, "Step Sizes(mm)"=w358, "IDs"=w360) -> ("error out"=w362:errorcluster)  [unwired: 3 in, 1 out]
      }
      frame "Stop Motion" {
        w365 = TRUE ("Close")
        n194 = local read "IDs"() -> (w367:i32[])
        n195 = for {
          shift-right: [w373] -> w370
          shift-left: w368 -> [w372]
          tunnel: w367 -> [w371] mode=indexing
          n196 = call "command stop.vi"("error in (no error)"=w372, "id"=w371) -> ("error out"=w373:errorcluster)  [unwired: 8 in, 1 out]
        }
        n197 = call "CloseDevices.vi"("error in (no error)"=w370, "Close"=w365, "Ids"=w367) -> ("error out"=w369:errorcluster)  [unwired: 8 in]
        n198 = local write "Moving?"(FALSE ("Moving?")) -> ()
      }
      frame "CloseApplication" {
        w374 = TRUE ("Close")
        n199 = local read "IDs"() -> (w377:i32[])
        n200 = for {
          shift-right: [w383] -> w380
          shift-left: w378 -> [w382]
          tunnel: w377 -> [w381] mode=indexing
          n201 = call "command stop.vi"("error in (no error)"=w382, "id"=w381) -> ("error out"=w383:errorcluster)  [unwired: 8 in, 1 out]
        }
        n202 = call "CloseDevices.vi"("error in (no error)"=w380, "Close"=w374, "Ids"=w377) -> ("error out"=w379:errorcluster)  [unwired: 8 in]
        n203 = local write "Moving?"(FALSE ("Moving?")) -> ()
      }
    }
    n204 = local read "Serial nos"() -> (w15:u32[])
    n205 = call <instrlib>:"Synchronous Latch.vi"("clear"=w23, "set"=w25) -> ("out"=w24:bool)  [unwired: 9 in]
    n206 = Not(x=w24) -> (.not. x?=w17:bool)
    n207 = Greater Than 0?(x=w15) -> (x > 0?=w14:bool[])
    n208 = Or(x=w29, y="Stop Stage") -> (x .or. y?=w26:bool)
    n209 = And Array Elements(Boolean array=w14) -> (logical AND=w13:bool)
    n210 = Select(t=StageOptions."Stop Motion", s=w26, f=w27) -> (s? t:f=w20:T6)
    n211 = And(x=w13, y=w17) -> (x .and. y?=→"Controller Open?":bool)
    n212 = Select(t=StageOptions."CloseApplication", s="Close Stage", f=w20) -> (s? t:f=w21:T6)
    "Stage Status" <- w32
  }
  n213 = while {
    shift-right: [w392] -> _
    shift-left: Generator_States."Idle" -> [w395]
    shift-right: [w393] -> _
    shift-left: errorcluster {"status"=FALSE, "code"=0, "source"=""} ("error in") -> [w394]
    stop <- w384 stop-if-true
    n214 = case shown="\"InitGen\"" w395 {
      tunnel: [w397 Generator_States."InitGen" Generator_States."Idle" Generator_States."Idle" Generator_States."Idle" Generator_States."Idle"] -> w391
      tunnel: w394 -> [w396 w411 w424 w430 w435 w442]
      tunnel: [w396 w405 w415 w429 w434 w441] -> w393
      tunnel: [_ _ TRUE ("Ext/nViTrig") _ _ _] -> w389
      tunnel: [_ _ _ _ TRUE ("x .or. y?") w438] -> w388
      tunnel: [_ _ _ _ _ w438] -> w384
      frame "Idle", Default {
        n215 = event shown="[3] \"Start Gen\": Value Change" {
          selector: _ -> [_ _ _ _]
          dyn-events: _ -> [_ _ _ _]
          timeout: 100 -> [_ _ _ _]
          tunnel: [Generator_States."Idle" Generator_States."SendVITrig" Generator_States."CloseGen" Generator_States."GenerateWaveArray"] -> w397
          event Timeout {
            n216 = event-data() -> ()  [unwired: 1 in, 3 out]
          }
          event "Send vi Trig": Value Change {
            n217 = event-data() -> ()  [unwired: 1 in, 6 out]
          }
          event "stop Gen": Value Change {
            n218 = event-data() -> ()  [unwired: 1 in, 6 out]
          }
          event "Start Gen": Value Change {
            n219 = event-data() -> ()  [unwired: 1 in, 6 out]
          }
        }
      }
      frame "GenerateWaveArray" {
        n220 = call "WaveSynthV2.vi"("error in"=w411, "Default Wave"="Use Default Wave Settings") -> ("error out"=w405:errorcluster, "Waves per Pixel 2"=→"Waves per Pixel":u32, "Sampling Frequency (Hz) 2"=→"Sampling Frequency (Hz)":u64, "Amplitudes"=→"Amplitudes" →"Input Waveform":dbl[], "Offset Factor 2"=→"Offset Factor":dbl, "Gain"=→"Gain":dbl)  [unwired: 2 in]
      }
      frame "InitGen" {
        n221 = local read "Gain"() -> (w419:dbl)
        n222 = local read "Amplitudes"() -> (w420:dbl[])
        n223 = local read "Sampling Frequency (Hz)"() -> (w422:u64)
        n224 = local read "Waves per Pixel"() -> (w421:u32)
        n225 = local read "Offset Factor"() -> (w418:dbl)
        n226 = call "InitGen.vi"("Offset"=w418, "Gain"=w419, "Ext/nViTrig"="Ext/nViTrig", "Waveform Data Array"=w420, "error in (no error)"=w424, "Wave Per Pixel"=w421, "Sample Rate (Samp/s)"=w422, "FGEN Resource Name"="Generator Resource") -> ("error out"=w416:errorcluster, "Actual Sample Rate"=→"Gen Actual Sample Rate":dbl, "reference out"=w414:refnum<k15>)  [unwired: 1 in]
        n227 = call "EnableOutput.vi"("error in (no error)"=w416, "FGEN Resource Name"=w414) -> ("error out"=w415:errorcluster)  [unwired: 8 in, 1 out]
      }
      frame "SendVITrig" {
        n228 = local read "Generator Resource"() -> (w426:refnum<k15>)
        n229 = call "SendTrig.vi"("error in (no error)"=w430, "Send vi Trig"="Send vi Trig", "Instrument Handle"=w426) -> ("error out"=w429:errorcluster)  [unwired: 7 in, 1 out]
      }
      frame "CloseGen" {
        n230 = local read "Generator Resource"() -> (w433:refnum<k15>)
        n231 = call "DisableOutput.vi"("error in (no error)"=w435, "FGEN Resource Name"=w433) -> ("error out"=w437:errorcluster, "Instrument Handle Out"=w436:refnum<k15>)  [unwired: 8 in]
        n232 = call "CloseGen.vi"("error in (no error)"=w437, "Instrument Handle"=w436) -> ("error out"=w434:errorcluster)  [unwired: 9 in]
      }
      frame "CloseApp" {
        w438 = TRUE ("x .or. y?")
        n233 = local read "Generator Resource"() -> (w440:refnum<k15>)
        n234 = call "DisableOutput.vi"("error in (no error)"=w442, "FGEN Resource Name"=w440) -> ("error out"=w444:errorcluster, "Instrument Handle Out"=w443:refnum<k15>)  [unwired: 8 in]
        n235 = call "CloseGen.vi"("error in (no error)"=w444, "Instrument Handle"=w443) -> ("error out"=w441:errorcluster)  [unwired: 9 in]
      }
    }
    n236 = call <instrlib>:"Synchronous Latch.vi"("clear"=w388, "set"=w389) -> ("out"=→"Generator On":bool)  [unwired: 9 in]
    n237 = Or(x="Stop Generator \nApplication", y=w393) -> (x .or. y?=w385:bool)
    n238 = Select(t=Generator_States."CloseApp", s=w385, f=w391) -> (s? t:f=w392:T1)
    "Gen State" <- w395
  }
  n239 = while {
    shift-right: [w454] -> _
    shift-left: Digitizer_StatesMain."Idle" -> [w459]
    shift-right: [w449] -> _
    shift-left: errorcluster {"status"=FALSE, "code"=0, "source"=""} ("error out") -> [w458]
    i -> [w456]
    stop <- w455 stop-if-true
    n240 = case shown="\"Read\"" w459 {
      tunnel: w458 -> [w476 w483 w500 w528 w558 w566]
      tunnel: [w476 w482 w502 w524 w557 w565] -> w449
      tunnel: [w475 Digitizer_StatesMain."SetParam" Digitizer_StatesMain."Read" Digitizer_StatesMain."Read" Digitizer_StatesMain."Idle" Digitizer_StatesMain."Idle"] -> w450
      tunnel: [_ _ _ _ _ w562] -> w455
      tunnel: [_ _ _ _ TRUE ("stop") w562] -> w447
      tunnel: [_ _ w495 _ _ _] -> w446
      frame "Idle", Default {
        n241 = Select(t=Digitizer_StatesMain."Init", s="Start Digi", f=Digitizer_StatesMain."Idle") -> (s? t:f=w475:T3)
      }
      frame "Init" {
        n242 = call "GetDigiRef.vi"("error in (no error)"=w483, "RIO Device IN"="Digi RIO Resource") -> ("error out"=w485:errorcluster, "FPGA VI Reference Out"=w478:T2)  [unwired: 8 in]
        n243 = disable-structure shown="Enabled" {
          disable-tunnel: w478 -> [w492 w493]
          disable-tunnel: [w491 w493] -> w477
          frame Disabled {
            n244 = xnode "Invoke Method"("FPGA VI Reference In"=w492) -> ("FPGA VI Reference Out"=w491:T2)  [unwired: 1 in, 1 out]
          }
          frame Enabled {
          }
        }
        n245 = call "InitDigitizer.vi"("error in"=w485, "FPGA VI Reference In"=w477) -> ("error out"=w488:errorcluster, "range (Vpp)"=→"range (Vpp)":dbl, "FPGA VI Reference Out"=w487:T10, "TIS Configured?"=→"TIS Configured?":bool, "Configured?"=→"Configured?":bool)  [unwired: 5 in]
        n246 = call "PXITrigReserve-Unreserve.vi"("error in"=w488, "Mode"=enum16{"Reserve", "Unreserve"}."Reserve", "FPGA VI Reference In"=w487) -> ("error out"=w482:errorcluster, "FPGA VI Reference Out"=→"FPGA VI Reference Out":T10)  [unwired: 7 in]
      }
      frame "SetParam" {
        w494 = i16 2000 ("WaveSampleCount")
        w495 = TRUE ("Arm?")
        n247 = local read "FPGA VI Reference Out"() -> (w499:T2)
        n248 = local read "range (Vpp)"() -> (w498:dbl)
        n249 = Power Of 2(x="Time Division") -> (2^x=w510:dbl)
        n250 = To Word Integer(number=w510) -> (16bit integer=w503:i16)
        "TimeDivFactor" <- w503
        n251 = call "ConfigAquisitionParam.vi"("Requested Samples Per Pixel"=sgl 200000000.0 ("Wave Sampling Rate"), "Downsample [0,1,2]"=w503, "ProcessCompletionDelay (us)"=w494, "vi/nGenTrig"="nGenTrig/vi", "error in"=w500, "AvgCount_powerOf2"="Amplitude \nAveraging", "Delay (us)"="Delay(us)", "FPGA VI Reference In"=w499) -> ("error out"=w515:errorcluster, "FPGA VI Reference Out"=w516:T10)  [unwired: 1 in, 1 out]
        n252 = call "TrigConfig.vi"("Trigger Level (V)"="Trigger Level (V)", "range (Vpp)"=w498, "error in"=w515, "Trigger Type"="Trigger Type", "Requested Samples Per Pixel"="Record Size", "FPGA VI Reference"=w516) -> ("error out"=w508:errorcluster, "Read Size (Host)"=→"Read Size (Host)":u16, "FPGA VI Reference Out"=w509:T2)  [unwired: 3 in]
        n253 = call "Arm(CommitSettings).vi"("Arm?"=w495, "error in"=w508, "FPGA VI Reference In"=w509) -> ("error out"=w502:errorcluster, "FPGA VI Reference Out"=w496:T10)  [unwired: 7 in]
        n254 = local write "FPGA VI Reference Out"(w496) -> ()
        "AvgCount_powerOf2" <- "Amplitude \nAveraging"
        "WaveSampleCount" <- w494
      }
      frame "Read" {
        n255 = local read "FPGA VI Reference Out"() -> (w522:T2)
        n256 = local read "Read Size (Host)"() -> (w526:u16)
        n257 = xnode "Read/Write Control"("FPGA VI Reference In"=w522) -> ("FPGA VI Reference Out"=w521:T2, "Trig out"=→"Trigger Count":u32, "Trig In"=→"Trig In":u32)  [unwired: 1 in, 1 out]
        n258 = Not(x="TrigIn_Sim") -> (.not. x?=w536:bool)
        n259 = call "ViTrig.vi"("Vi Trigger"=w536, "error in"=w528, "FPGA VI Reference In"=w521) -> ("error out"=w532:errorcluster, "FPGA VI Reference Out"=w531:T10)  [unwired: 7 in]
        n260 = call "ReadFromDigi.vi"("Timeout (ms)"=200, "error in"=w532, "Number of Elements"=w526, 10:enum16{"Wait For Data", "Timeout"}."Timeout" ("Mode"), "FPGA VI Reference In"=w531) -> ("error out"=w525:errorcluster, "Data Valid?"=w535:bool, "Output Waveform"=w533:u16[])  [unwired: 3 in, 1 out]
        n261 = case shown="False" w535 {
          tunnel: w533 -> [w538 _]
          tunnel: w525 -> [w540 w553]
          tunnel: [w539 w553] -> w524
          tunnel: [TRUE ("increment") _] -> w519
          frame False {
            n262 = local read "TimeDivFactor"() -> (w541:i16)
            n263 = local read "Delay(us)"() -> (w543:sgl)
            n264 = local read "range (Vpp)"() -> (w542:dbl)
            n265 = Divide(x=1600000000.0 ("Sample Rate"), y=w541) -> (x/y=w545:dbl)
            n266 = disable-structure shown="Disabled" {
              disable-tunnel: w540 -> [w551 w552]
              disable-tunnel: [w550 w552] -> w539
              disable-tunnel: w538 -> [w549 _]
              frame Disabled {
                n267 = call "ReadDataQueue.vi"("Write/nRead"=FALSE, "error in (no error)"=w551, "Output Waveform"=w549) -> ("error out"=w550:errorcluster)  [unwired: 7 in, 1 out]
              }
              frame Enabled {
              }
            }
            n268 = call "Scale Acquired Data.vi"("range (V)"=w542, "Start Time (us)"=w543, "Sample Rate"=w545, "Number of Bits"=i16 16, "Data In"=w538) -> ("output waveform"=→"Waveform LIVE":cluster{"Start Time":dbl, dbl, ext[]})  [unwired: 6 out]
          }
          frame True {
          }
        }
        n269 = call-poly <instrlib>:"Count Up.vi"("increment"=w519, "reset"="reset") -> ("count out"=→"count out":u32)  [unwired: 13 in]
      }
      frame "CloseDigi" {
        n270 = local read "FPGA VI Reference Out"() -> (w556:T2)
        n271 = call "PXITrigReserve-Unreserve.vi"("error in"=w558, "Mode"=enum16{"Reserve", "Unreserve"}."Unreserve", "FPGA VI Reference In"=w556) -> ("error out"=w561:errorcluster, "FPGA VI Reference Out"=w560:T10)  [unwired: 7 in]
        n272 = xnode "Close FPGA VI Reference"("FPGA VI Reference In"=w560, "error in"=w561) -> ("error out"=w557:errorcluster)
      }
      frame "CloseApp" {
        w562 = TRUE ("stop")
        n273 = local read "FPGA VI Reference Out"() -> (w564:T2)
        n274 = call "PXITrigReserve-Unreserve.vi"("error in"=w566, "Mode"=enum16{"Reserve", "Unreserve"}."Unreserve", "FPGA VI Reference In"=w564) -> ("error out"=w569:errorcluster, "FPGA VI Reference Out"=w568:T10)  [unwired: 7 in]
        n275 = xnode "Close FPGA VI Reference"("FPGA VI Reference In"=w568, "error in"=w569) -> ("error out"=w565:errorcluster)
      }
    }
    n276 = event shown="[4] \"FineDelay  Control\": Value Change" {
      selector: _ -> [_ _ _ _ _]
      dyn-events: _ -> [_ _ _ _ _]
      timeout: 0 -> [_ _ _ _ _]
      event "Delay(us)": Value Change {
        w464 = 0.1 ("Scale.Range:Increment")
        n277 = event-data() -> ("NewVal"=w461:sgl)  [unwired: 1 in, 5 out]
        n278 = Subtract(x=w461, y="Range") -> (x-y=w463:dbl)
        n279 = Add(x=w461, y="Range") -> (x+y=w462:dbl)
        n280 = property on="FineDelay  Control" class="Slide (strict)"("Scale.Increment"=w464, "Scale.MinorInc"=w464, "Scale.Minimum"=w463, "Scale.Maximum"=w462, "Value"=w461) -> ()  [unwired: 2 in, 2 out]
      }
      event "Amplitude Range": Value Change {
        n281 = event-data() -> ("NewVal"=w467:cluster{"Slider 1":dbl, "Slider 1":dbl})  [unwired: 1 in, 5 out]
        n282 = Unbundle(w467) -> ("Slider 1"=w465:dbl, "Slider 1"=w466:dbl)
        n283 = property on="Waveform LIVE" class="WFGraph (strict)"("YScale.Maximum"=w466, "YScale.Minimum"=w465) -> ()  [unwired: 2 in, 2 out]
      }
      event Timeout {
        n284 = event-data() -> ()  [unwired: 1 in, 3 out]
      }
      event "Start Digi": Value Change {
        n285 = event-data() -> ()  [unwired: 1 in, 6 out]
      }
      event "FineDelay  Control": Value Change {
        n286 = event-data() -> ("NewVal"=w469:dbl)  [unwired: 1 in, 5 out]
        n287 = property on="Delay(us)" class="DigNum (strict)"() -> ("Value"=w470:sgl)  [unwired: 2 in, 2 out]
        n288 = Add(x=w469, y=w470) -> (x+y=w468:dbl)
        n289 = property on="Delay(us)" class="DigNum (strict)"("Value"=w468) -> ()  [unwired: 2 in, 2 out]
      }
    }
    n290 = Equal To 0?(x=w456) -> (x = 0?=w457:bool)
    n291 = case shown="True" w457 {
      frame False {
      }
      frame True {
        n292 = property on="Delay(us)" class="DigNum (strict)"("Val(Sgnl)"=sgl 0.0 ("Value (Signaling)")) -> ()  [unwired: 2 in, 2 out]
      }
    }
    n293 = call <instrlib>:"Synchronous Latch.vi"("clear"=w447, "set"=w446) -> ("out"=→"Digitizer On":bool)  [unwired: 9 in]
    n294 = Or(x="Stop Digi App", y=w449) -> (x .or. y?=w451:bool)
    n295 = Select(t=Digitizer_StatesMain."CloseApp", s=w451, f=w450) -> (s? t:f=w454:T3)
    "Digi State" <- w459
  }
  n296 = while {
    shift-right: [w584] -> _
    shift-left: w3 -> [w587]
    shift-right: [w585] -> _
    shift-left: _ -> [w586]
    shift-right: [w583] -> _
    shift-left: ScanStates_main."Idle" -> [w588]
    shift-right: [w582] -> _
    shift-left: w4 -> [w581]
    shift-right: [w579] -> _
    shift-left: w2 -> [w580]
    shift-right: [w578] -> _
    shift-left: w5 -> [w575]
    shift-right: [w577] -> _
    shift-left: w6 -> [w576]
    shift-right: [w573] -> _
    shift-left: _ -> [w572]
    shift-right: [w571] -> _
    shift-left: _ -> [w570]
    stop <- FALSE stop-if-true
    n297 = case shown="\"Init\"" w588 {
      tunnel: w587 -> [w600 _ w868 w884 w908]
      tunnel: w586 -> [w599 _ w871 w885 w906]
      tunnel: [w599 w625 w870 w885 w906] -> w585
      tunnel: [w600 w602 w868 w884 w908] -> w584
      tunnel: [w596 ScanStates_main."Get Data" ScanStates_main."Store Data" ("f") w882 ScanStates_main."Idle" ("f")] -> w583
      tunnel: [w591 i16[] [] ("Waveform") w869 w873 w905] -> w582
      tunnel: w581 -> [w591 _ _ w873 w905]
      tunnel: w580 -> [w592 _ w867 w883 w907]
      tunnel: [w592 u64 0 ("Point Counter") w866 w883 w907] -> w579
      tunnel: [w593 w603 w853 w878 w903] -> w578
      tunnel: [w594 w601 w861 w879 w904] -> w577
      tunnel: w576 -> [w594 _ w863 w879 w904]
      tunnel: w575 -> [w593 _ w862 w878 w903]
      tunnel: [w590 w614 w855 w877 w899] -> w573
      tunnel: w572 -> [w590 _ w855 w877 w901]
      tunnel: [w589 w615 w854 w875 w898] -> w571
      tunnel: w570 -> [w589 _ w854 w876 w900]
      frame "Idle", Default {
        n298 = Select(t=ScanStates_main."Init", s="Start Scan", f=ScanStates_main."Idle") -> (s? t:f=w596:T7)
      }
      frame "Init" {
        n299 = flat-sequence {
          tunnel: [w834] -> w603
          tunnel: [w833] -> w602
          tunnel: [w832] -> w601
          tunnel: [w844] -> w624
          tunnel: [w848] -> w625
          tunnel: w624 -> [w848]
          frame #0 {
            n300 = while {
              stop <- w829 stop-if-true
              n301 = local read "Generator On"() -> (w829:bool)
              n302 = Not(x=w829) -> (.not. x?=w828:bool)
              n303 = local write "Start Gen"(w828) -> ()
            }
          }
          frame #1 {
            n304 = while {
              stop <- w831 stop-if-true
              n305 = local read "Digitizer On"() -> (w831:bool)
              n306 = Not(x=w831) -> (.not. x?=w830:bool)
              n307 = local write "Start Digi"(w830) -> ()
            }
          }
          frame #2 {
            w840 = sgl 0.0 ("X Start")
            n308 = local read "Pixel Count"() -> (w835:i32)
            n309 = local read "Line Count"() -> (w836:i32)
            n310 = local read "Scan Mode"() -> (w843:enum16{"Raster", "Serpentine"})
            n311 = Decrement(x=w836) -> (x-1=w841:i32)
            n312 = Decrement(x=w835) -> (x-1=w842:i32)
            n313 = Initialize Array(0.0 ("element"), w836, w835) -> (w832:dbl[][])
            n314 = Initialize Array(0.0 ("element"), w836, w835) -> (w834:dbl[][])
            n315 = call "GenerateScanEndPts.vi"("X Start"=w840, "Mode"=w843, "X End"=w842, "Y Start"=w840, "Y End"=w841, "Line Count"=w836, "Pixel Count"=w835, "EdgePt/nPixelMap"=FALSE) -> ("Coordinate Array"=w833:sgl[][])  [unwired: 3 in, 4 out]
          }
          frame #3 {
            n316 = Obtain Queue(name (unnamed)="AquiredDataFIFO", element data type=i16[] [] ("16bit integer"), create if not found? (T)=TRUE) -> (queue out=w844:refnum<queue>)  [unwired: 2 in, 2 out]
          }
          frame #4 {
            n317 = while {
              stop <- w850 stop-if-true
              n318 = local read "Machine Mode"() -> (w852:T4)
              n319 = Equal?(x=w852, y=T4."Scanning Mode") -> (x = y?=w850:bool)
              n320 = Not(x=w850) -> (.not. x?=w849:bool)
              n321 = local write "Start Stage"(w849) -> ()
            }
          }
        }
        n322 = Get Date/Time In Seconds() -> (seconds since 1Jan1904=w606:timestamp)
        n323 = Format Date/Time String(time format string (%c)="(%d-%m-%y %H-%M-%S).h5", seconds (now)=w606) -> (date/time string=w605:string)  [unwired: 1 in]
        n324 = Concatenate Strings("Filename", w605) -> (w608:string)
        n325 = String To Path(string=w608) -> (path=w610:path)
        n326 = Build Path(base path="File Directory", name or relative path=w610) -> (appended path=w604:path)
        n327 = call <vilib>:"OpenCreateReplace HDF5 File.vi"("function (open or create)"=LVH5F_Operation."create or replace (with confirmation)", "path"=w604) -> ("error out"=w613:errorcluster, "HDF5 Ref out"=w616:T17)  [unwired: 6 in]
        n328 = xnode "Simple H5Dwrite"("Dataset Path"="data", "Unlimited  dataset (F)"=TRUE, "error in (no error)"=w613, "operation (open or create)"=LVH5D_Operation."create or replace with confirmation", "HDF5 Path or Ref"=w616, "Data"=i16[][] [] ("Waveform")) -> ("HDF5 Dataset Ref out"=w615:T17, "HDF5 Ref out"=w614:T17)  [unwired: 2 in, 1 out]
        n329 = disable-structure shown="Disabled" {
          frame Disabled {
            n330 = call "OpenH5WithAttr.vi"() -> ()  [unwired: 10 in, 2 out]
          }
          frame Enabled {
          }
        }
      }
      frame "Get Data" {
        n331 = Dequeue Element(queue=w871) -> (queue out=w870:refnum<queue>, element=w869:i16[])  [unwired: 2 in, 2 out]
        n332 = Absolute Value(x=w869) -> (abs(x)=w864:i16[])
        n333 = Array Max & Min(array=w864) -> (max value=w860:i16, max index (indices)=w857:i32)  [unwired: 2 out]
        n334 = Index Array(array=w868, index (row)=w867) -> (element=w865:sgl[])  [unwired: 1 in]
        n335 = Index Array(array=w865) -> (element #1=w859:sgl, element #2=w858:sgl)  [unwired: 2 in]
        n336 = Increment(x=w867) -> (x+1=w866:u64)
        n337 = Replace Array Subset(array=w862, new element=w860, index (row)=w859, index (col)=w858) -> (w853:dbl[][])
        "Intensity Graph" <- w853
        n338 = Replace Array Subset(array=w863, new element=w857, index (row)=w859, index (col)=w858) -> (w861:dbl[][])
      }
      frame "Store Data" {
        n339 = Build Array(w873) -> (w872:i16[][])
        n340 = xnode "Append Element(s) to Dataset"("Dimension to Extend (0)"=0, "HDF5 Dataset Ref"=w876, "Data Element(s)"=w872) -> ("HDF5 Dataset out"=w875:T17)  [unwired: 1 in, 3 out]
        n341 = Matrix Size(0:w884) -> (1:w887:i32)  [unwired: 1 out]
        n342 = Greater?(x=w883, y=w887) -> (0:w886:bool)
        n343 = Select(t=ScanStates_main."Close Files", s=w886, f=ScanStates_main."Get Data") -> (s? t:f=w882:T7)
      }
      frame "Close Files" {
        w898 = T17 refnum items=["HDF5 Ref"] ("HDF5 Dataset out")
        w899 = T17 refnum items=["HDF5 Ref"] ("HDF5 Ref out")
        n344 = call <vilib>:"H5Dclose.vi"("HDF5 Dataset Ref"=w900) -> ("error out"=w897:errorcluster)  [unwired: 8 in]
        n345 = call <vilib>:"H5Fclose.vi"("error in (no error)"=w897, "Force Close (F)"=TRUE, "HDF5 Ref"=w901) -> ()  [unwired: 6 in, 1 out]
      }
    }
  }
